vi "Pixels per frame.vi"(10 "Rising edge":bool, 11 ">> # of pixels collected in a frame >>":u32) -> (2 "samples acquired":u32, 3 "Boolean out":bool)   [LabVIEW 2015]
uses:
  <vilib>/rvi/Emulation/niFpgaSctlEmulationGetInTimedLoop.vi
  Globals/Global_Sample per Frame.vi
  <vilib>/rvi/Emulation/niFpgaProcessEmulError.vi
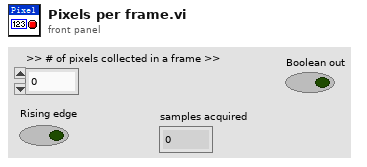
[diagram p1: front panel]
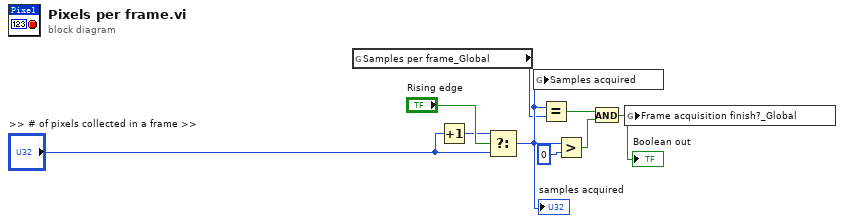
[diagram p0: block diagram]
diagram:
  n1 = global read "Global_Sample per Frame.vi" "Samples per frame_Global"() -> (w8:u32)
  n2 = Increment(x=">> # of pixels collected in a frame >>") -> (x+1=w6:u32)
  n3 = Select(t=w6, s="Rising edge", f=">> # of pixels collected in a frame >>") -> (s? t:f=w9:u32)
  "samples acquired" <- w9
  n4 = global write "Global_Sample per Frame.vi" "Samples acquired"(w9) -> ()
  n5 = Equal?(x=w9, y=w8) -> (x = y?=w5:bool)
  n6 = Greater?(x=w9, y=u32 0) -> (0:w4:bool)
  n7 = And(x=w5, y=w4) -> (x .and. y?=w1:bool)
  "Boolean out" <- w1
  n8 = global write "Global_Sample per Frame.vi" "Frame acquisition finish?_Global"(w1) -> ()
